vi "角度转换到-90到90.vi"(11 "数值输入":dbl) -> (3 "数值输出":dbl)   [LabVIEW 2014]
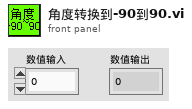
[diagram p1: front panel]
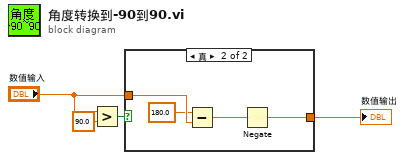
[diagram p0: block diagram]
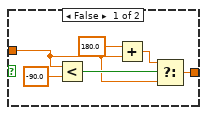
[diagram p2: hidden frame]
diagram:
  n1 = Greater?(x="数值输入", y=90.0) -> (0:w2:bool)
  n2 = case shown="真" w2 {
    tunnel: "数值输入" -> [w6 w14]
    tunnel: [w8 w11] -> w4
    frame False {
      n3 = Less?(x=w6, y=-90.0) -> (x < y?=w9:bool)
      n4 = Add(x=180.0, y=w6) -> (x+y=w7:dbl)
      n5 = Select(t=w7, s=w9, f=w6) -> (s? t:f=w8:dbl)
    }
    frame True {
      n6 = Subtract(x=180.0, y=w14) -> (x-y=w12:dbl)
      n7 = Negate(x=w12) -> (-x=w11:dbl)
    }
  }
  "数值输出" <- w4
